vi "hardware_close_hardware.vi"(8 "error in (no error)":errorcluster, 11 "picoquant_generic in":refnum<class "picoquant_generic.lvclass">) -> (0 "error out":errorcluster, 3 "picoquant_generic out":refnum<class "picoquant_generic.lvclass">)   [LabVIEW 2015, in "picoquant_generic.lvclass"]
uses:
  picoquant_generic.lvclass
  detector/detector.lvclass
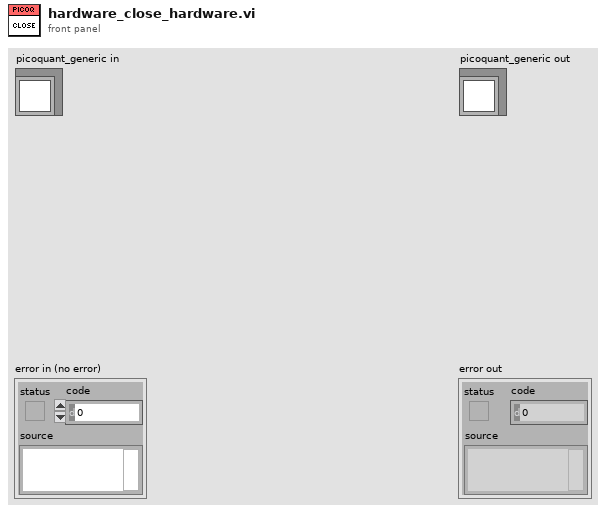
[diagram p1: front panel]
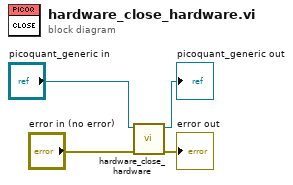
[diagram p0: block diagram]
diagram:
  n1 = call-parent "hardware_close_hardware.vi"("error in (no error)"="error in (no error)", "hardware in"="picoquant_generic in") -> ("error out"=→"error out":errorcluster, "hardware out"=→"picoquant_generic out":refnum<class "picoquant_generic.lvclass">)  [unwired: 8 in]
